vi "UDP_Test.vi"() -> ()   [LabVIEW 2016]
uses:
  SerialSupport/Serial - Settings.ctl
  SerialSupport/Serial - XON-XOFF Characters.ctl
  SerialSupport/Serial - ASCII Characters.ctl
  <vilib>/Instr/_visa.llb/VISA Configure Serial Port (Instr).vi
panel:
  in  "Stop":bool
  in  "Serial out":string caption="字符串输出"
  out "读取缓冲区":string
  in  "终止符":u8=10 format="%.0x"
  in  "终止符时结束写入？":bool=TRUE
  in  "VISA资源名称":refnum<visa-resource-name>="COM1"
  in  "XON/XOFF字符":T1={"XON"=enum."DC1", "XOFF"=enum."DC3"}
  in  "串口设置":T3={"波特率"=115200, "数据位"=8, "校验"=enum."None", "停止位"=10, "流控制"=0} {"流控制" items=["无"=0, "XON/XOFF"=1, "RTS/CTS"=2, "DTR/DSR"=4]; "停止位" items=["1.0"=10, "1.5"=15, "2.0"=20]; "数据位" min=5 max=8 step=1; "波特率" items=["75"=75, "110"=110, "134"=134, "150"=150, "300"=300, "600"=600, "1200"=1200, "1800"=1800, "2400"=2400, "4800"=4800, "7200"=7200, "9600"=9600, "14400"=14400, "19200"=19200, "28800"=28800, "38400"=38400, "56000"=56000, "57600"=57600, "115200"=115200, "128000"=128000, "230400"=230400]}
  in  "终止符时结束读取？":bool=TRUE
  out "响应":string
  in  "读数":u32=1000
  in  "读取":bool
  in  "停止 2":bool
  in  "x":dbl
  in  "string out":string caption="字符串输出"
  in  "停止":bool
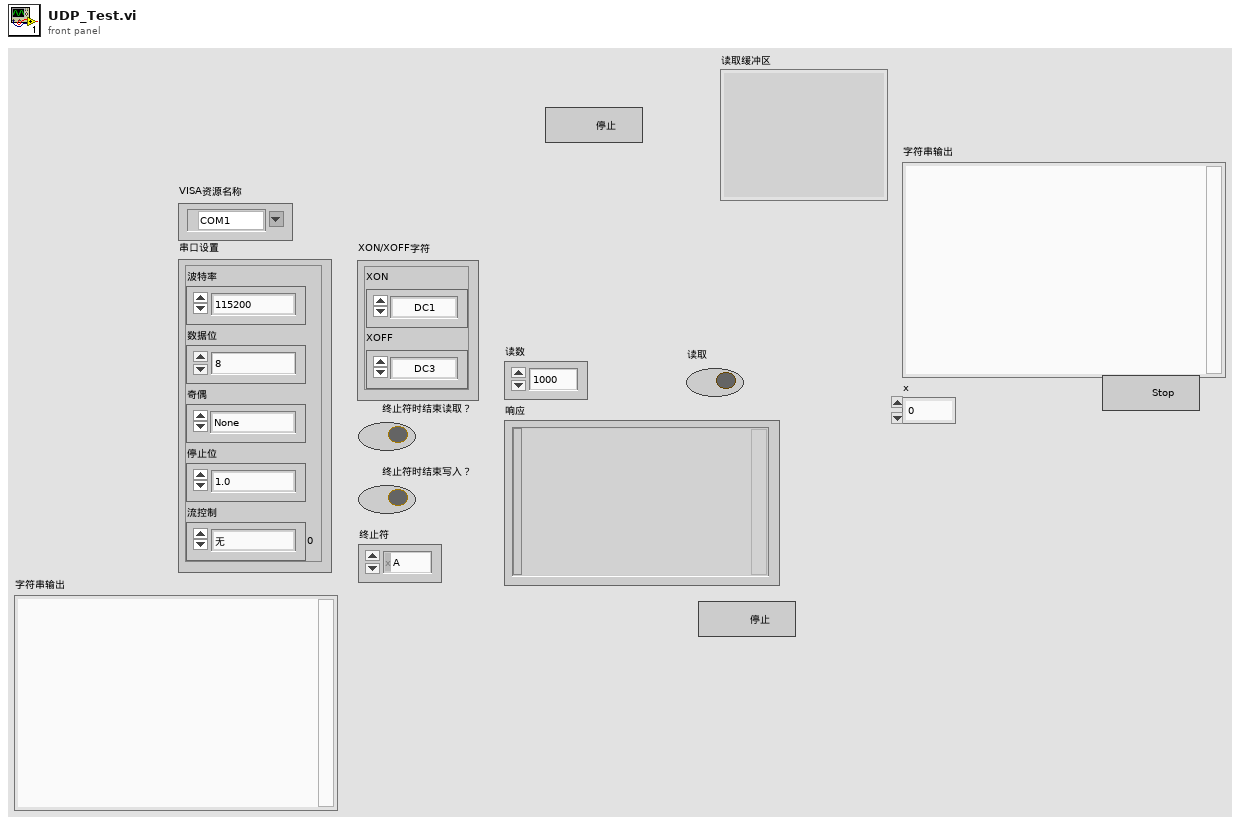
[diagram p1: front panel]
types:
  T1 = typedef "Serial - XON-XOFF Characters.ctl" = cluster{"XON":T2, "XOFF":T2}
  T2 = typedef "Serial - ASCII Characters.ctl" = enum16{"NUL", "SOH", "STX", "ETX", "EOT", "ENQ", "ACK", "BEL", "BS", "HT", "LF", "VT", "FF", "CR", "SO", "SI", "DLE", "DC1", "DC2", "DC3", "DC4", "NAK", "SYN", "ETB", "CAN", "EM", "SUB", "ESC", "FS", "GS", "RS", "US", "SP", "!", "\"", "#", "$", "%", "&", "'", "(", ")", "*", "+", ",", "- (-)", ".", "/", "0", "1", "2", "3", "4", "5", "6", "7", "8", "9", ":", ";", "<", "=", ">", "?", "@", "A", "B", "C", "D", "E", "F", "G", "H", "I", "J", "K", "L", "M", "N", "O", "P", "Q", "R", "S", "T", "U", "V", "W", "X", "Y", "Z", "[", "\\", "]", "^", "_", "`", "a", "b", "c", "d", "e", "f", "g", "h", "i", "j", "k", "l", "m", "n", "o", "p", "q", "r", "s", "t", "u", "v", "w", "x", "y", "z", "{", "|", "}", "~"}
  T3 = typedef "Serial - Settings.ctl" = cluster{"波特率":u32, "数据位":u16, "校验":enum16{"None", "Odd", "Even", "Mark", "Space"}, "停止位":u16, "流控制":u16}
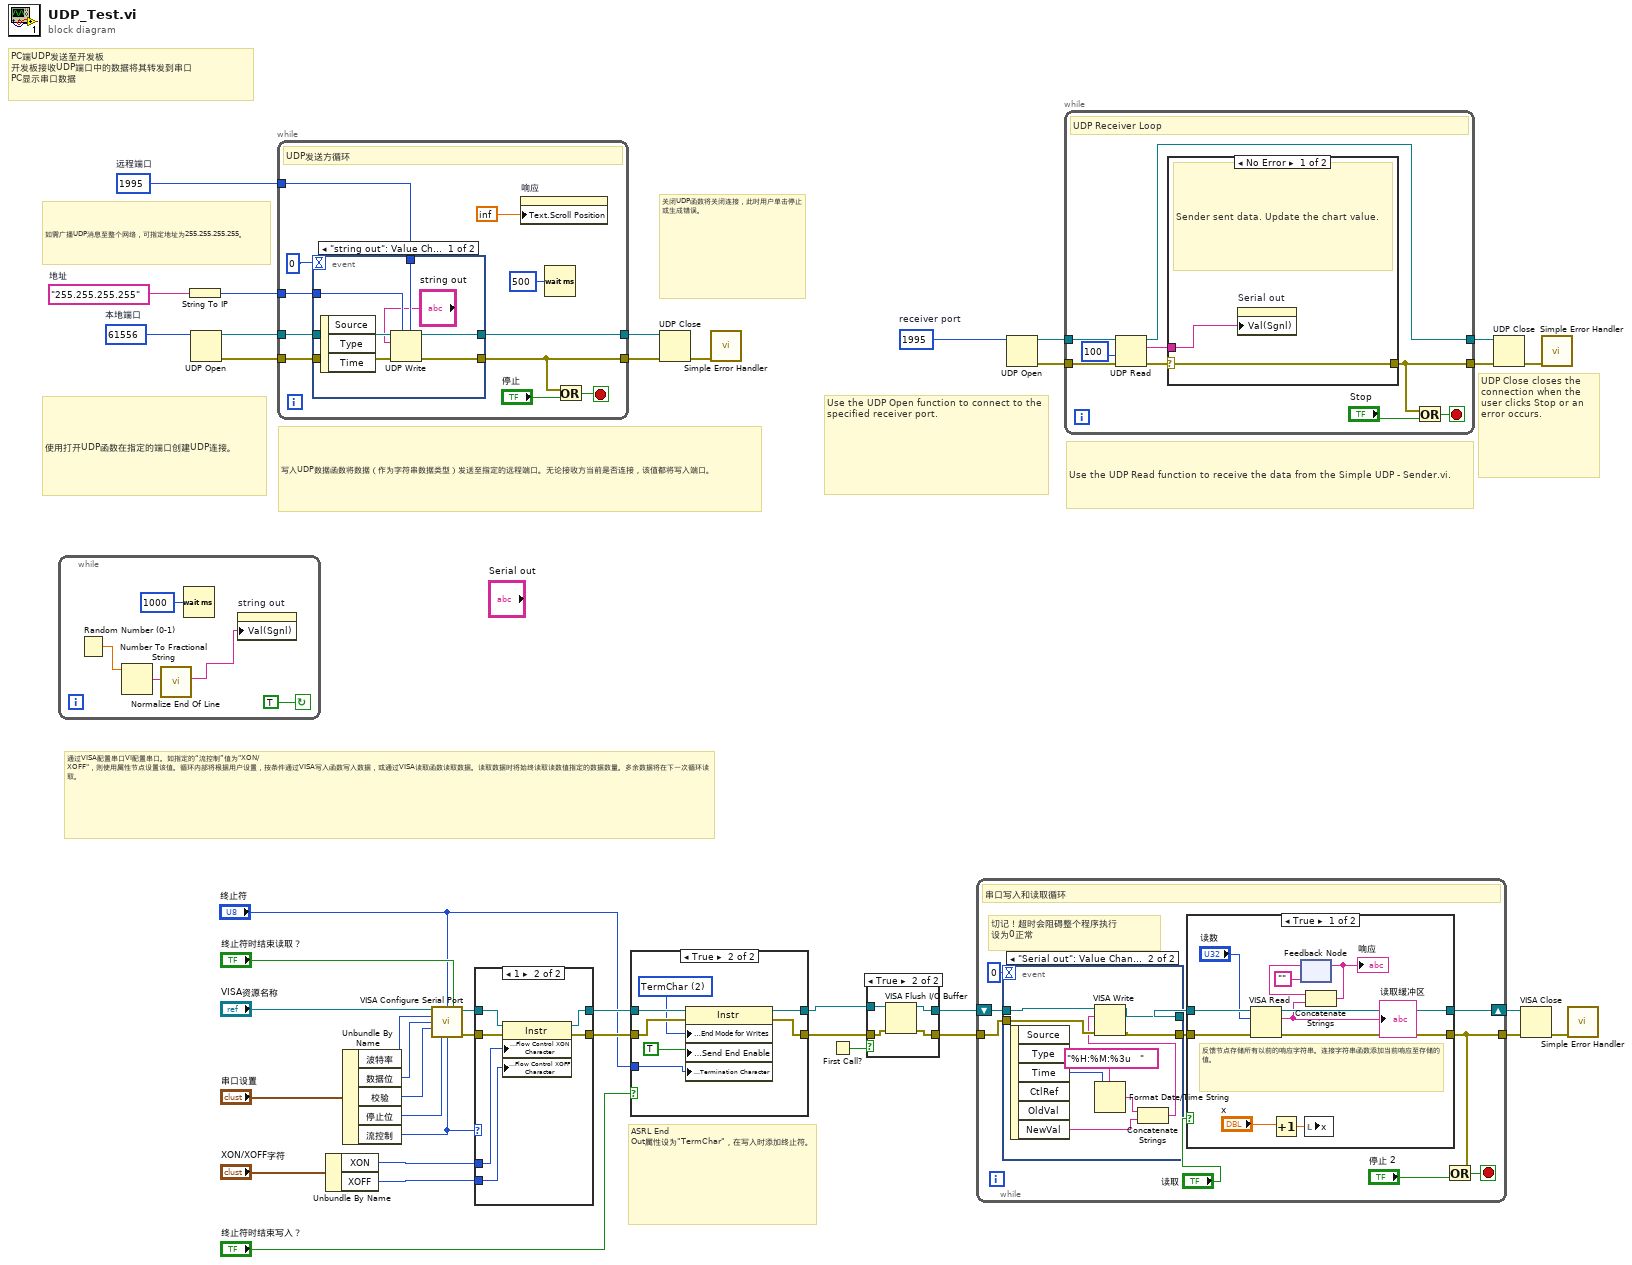
[diagram p0: block diagram]
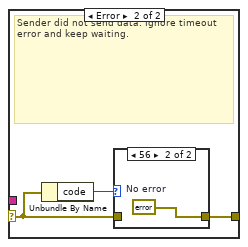
[diagram p2: hidden frame]
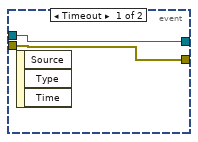
[diagram p7: hidden frame]
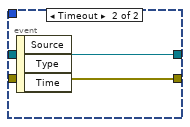
[diagram p9: hidden frame]
diagram:
  w6 = u16 1995  # receiver port
  w32 = u16 1995  # 远程端口
  w33 = u16 61556  # 本地端口
  w38 = "255.255.255.255"  # 地址
  # "UDP Close closes the connection when the user clicks Stop or an error occurs."
  # "Use the UDP Open function to connect to the specified receiver port."
  # "Use the UDP Read function to receive the data from the Simple UDP - Sender.vi."
  # "PC端UDP发送至开发板\n开发板接收UDP端口中的数据将其转发到串口\nPC显示串口数据"
  # "ASRL End Out属性设为\"TermChar\"，在写入时添加终止符。"
  # "通过VISA配置串口VI配置串口。如指定的“流控制”值为\"XON/XOFF\"，则使用属性节点设置该值。循环内部将根据用户设置，按条件通过VISA写入函数写入数据，或通过VISA读取函数读取数据。读取数据时将始终读取读数值指定的数据数量。多余数据将在下一次循环读取。"
  # "如需广播UDP消息至整个网络，可指定地址为255.255.255.255。"
  # "关闭UDP函数将关闭连接，此时用户单击停止或生成错误。"
  # "写入UDP数据函数将数据（作为字符串数据类型）发送至指定的远程端口。无论接收方当前是否连接，该值都将写入端口。"
  # "使用打开UDP函数在指定的端口创建UDP连接。"
  n1 = while {
    stop <- TRUE continue-if-true
    n2 = Random Number (0-1)() -> (number: 0 to 1=w44:dbl)
    n3 = Number To Fractional String(number=w44) -> (F-format string=w43:string)  [unwired: 3 in]
    n4 = call <vilib>:"Normalize End Of Line.vi"("string in"=w43) -> ("string out"=w41:string)  [unwired: 7 in]
    n5 = Wait (ms)(milliseconds to wait=u32 1000 ("等待时间（毫秒）")) -> ()  [unwired: 1 out]
    n6 = property on="string out" class="Str"("Val(Sgnl)"=w41) -> ()  [unwired: 2 in, 2 out]
  }
  n7 = String To IP(1:w38) -> (0:w36:u32)
  n8 = UDP Open(11:w33) -> (port=w35:refnum<k16>, 0:w34:errorcluster)  [unwired: 4 in, 1 out]
  n9 = while {
    tunnel: [w51] -> w39
    tunnel: w35 -> [w56]
    tunnel: w34 -> [w55]
    tunnel: [w52] -> w40
    tunnel: w36 -> [w50]
    tunnel: w32 -> [w48]
    stop <- w54 stop-if-true
    # "UDP发送方循环"
    n10 = event shown="[0] \"string out\": Value Change" {
      selector: _ -> [_ _]
      dyn-events: _ -> [_ _]
      timeout: 0 -> [_ _]
      tunnel: w56 -> [w63 w65]
      tunnel: w55 -> [w62 w64]
      tunnel: [w61 w65] -> w52
      tunnel: [w60 w64] -> w51
      tunnel: w50 -> [w59 _]
      tunnel: w48 -> [w58 _]
      event "string out": Value Change {
        n11 = event-data() -> ()  [unwired: 1 in, 3 out]
        n12 = UDP Write(address=w59, port or service name=w58, connection ID=w63, data in="string out", 8:w62) -> (error out=w60:errorcluster, 3:w61:refnum<k16>)  [unwired: 1 in]
      }
      event Timeout {
        n13 = event-data() -> ()  [unwired: 1 in, 3 out]
      }
    }
    n14 = property on="响应" class="Str"("Text.Scroll Position"=inf) -> ()  [unwired: 2 in, 2 out]
    n15 = Wait (ms)(milliseconds to wait=u32 500) -> ()  [unwired: 1 out]
    n16 = Or(x=w51, y="停止") -> (x .or. y?=w54:bool)
  }
  n17 = Unbundle By Name("XON/XOFF字符") -> ("XON"=w17:T2, "XOFF"=w16:T2)
  n18 = Unbundle By Name("串口设置") -> ("波特率"=w24:u32, "数据位"=w25:u16, "校验"=w26:enum16{"None", "Odd", "Even", "Mark", "Space"}, "停止位"=w27:u16, "流控制"=w18:u16)
  n19 = call-poly "VISA Configure Serial Port"("VISA resource name"="VISA资源名称", "termination char\n(0xA = '\\n' = LF)"="终止符", "Enable Termination\nChar (T)"="终止符时结束读取？", "baud rate (9600)"=w24, "data bits (8)"=w25, "parity (0:none)"=w26, "stop bits (10: 1 bit)"=w27, "flow control (0:none)"=w18) -> ("VISA resource name out"=w28:refnum<visa-resource-name>, "error out"=w29:errorcluster)  [unwired: 2 in, 4 out]
  n20 = case shown="1" w18 {
    tunnel: [w66 w73] -> w15
    tunnel: [w67 w72] -> w14
    tunnel: w29 -> [w66 w71]
    tunnel: w28 -> [w67 w70]
    tunnel: w17 -> [_ w69]
    tunnel: w16 -> [_ w68]
    frame Default {
    }
    frame 1 {
      n21 = property class="Instr"(reference=w70, error in=w71, "Serial Settings:Flow Control XON Character"=w69, "Serial Settings:Flow Control XOFF Character"=w68) -> (reference out=w72:refnum<visa-resource-name>, error out=w73:errorcluster)
    }
  }
  n22 = case shown="True" "终止符时结束写入？" {
    tunnel: w14 -> [w74 w82]
    tunnel: w15 -> [w75 w81]
    tunnel: [w74 w80] -> w11
    tunnel: [w75 w79] -> w10
    tunnel: "终止符" -> [_ w77]
    frame False {
    }
    frame True {
      w78 = u16 2 items=["None", "LastBit", "TermChar", "Break"] ("Serial Settings:Serial End Mode for Writes")
      n23 = property class="Instr"(reference=w82, error in=w81, "Serial Settings:End Mode for Writes"=w78, "Message Based Settings:Send End Enable"=TRUE, "Message Based Settings:Termination Character"=w77) -> (reference out=w80:refnum<visa-resource-name>, error out=w79:errorcluster)
    }
  }
  n24 = UDP Close(connection ID=w40, 8:w39) -> (error out=w37:errorcluster)  [unwired: 1 out]
  n25 = call <vilib>:"Simple Error Handler.vi"("error in (no error)"=w37) -> ()  [unwired: 4 in, 5 out]
  n26 = First Call?() -> (First Call?: T/F=w7:bool)
  n27 = case shown="True" w7 {
    tunnel: w11 -> [w84 w88]
    tunnel: w10 -> [w83 w87]
    tunnel: [w84 w86] -> w9
    tunnel: [w83 w85] -> w8
    frame False {
    }
    frame True {
      n28 = VISA Flush I/O Buffer(VISA resource name=w88, error in (no error)=w87) -> (VISA resource name out=w86:refnum<visa-resource-name>, error out=w85:errorcluster)  [unwired: 1 in]
    }
  }
  n29 = while {
    shift-right: [w98] -> w19
    shift-left: w9 -> [w91]
    tunnel: w8 -> [w93]
    tunnel: [w95] -> w20
    stop <- w96 stop-if-true
    # "切记！超时会阻碍整个程序执行\n设为0正常"
    # "串口写入和读取循环"
    n30 = event shown="[1] \"Serial out\": Value Change" {
      selector: _ -> [_ _]
      dyn-events: _ -> [_ _]
      timeout: 0 -> [_ _]
      tunnel: w93 -> [w99 w109]
      tunnel: [w99 w108] -> w92
      tunnel: w91 -> [w100 w107]
      tunnel: [w100 w106] -> w90
      event Timeout {
        n31 = event-data() -> ()  [unwired: 1 in, 3 out]
      }
      event "Serial out": Value Change {
        n32 = event-data() -> ("Time"=w105:u32, "NewVal"=w103:string)  [unwired: 1 in, 4 out]
        n33 = Format Date/Time String(time format string (%c)="%H:%M:%3u   " ("时间格式字符串(%c)"), seconds (now)=w105) -> (date/time string=w102:string)  [unwired: 1 in]
        n34 = Concatenate Strings(w102, w103) -> (w101:string)
        n35 = VISA Write(VISA resource name=w107, write buffer=w101, error in (no error)=w109) -> (VISA resource name out=w106:refnum<visa-resource-name>, error out=w108:errorcluster)  [unwired: 1 out]
      }
    }
    n36 = case shown="True" "读取" {
      tunnel: [w118 w122] -> w98
      tunnel: w90 -> [w120 w122]
      tunnel: [w116 w121] -> w95
      tunnel: w92 -> [w119 w121]
      frame True {
        # "反馈节点存储所有以前的响应字符串。连接字符串函数添加当前响应至存储的值。"
        n37 = VISA Read(VISA resource name=w120, byte count="读数", error in (no error)=w119) -> (VISA resource name out=w118:refnum<visa-resource-name>, read buffer=w115:string, error out=w116:errorcluster)  [unwired: 1 out]
        "读取缓冲区" <- w115
        n38 = Increment(x="x") -> (x+1=w110:dbl)
        n39 = feedback #1("") -> (w114:string)
        n40 = local write "x"(w110) -> ()
        n41 = Concatenate Strings(w114, w115) -> (w113:string)
        "响应" <- w113
        n42 = feedback-in #1(w113) -> ()
      }
      frame False {
      }
    }
    n43 = Or(x=w95, y="停止 2") -> (x .or. y?=w96:bool)
  }
  n44 = UDP Open(11:w6) -> (port=w5:refnum<k16>, 0:w4:errorcluster)  [unwired: 4 in, 1 out]
  n45 = while {
    tunnel: w5 -> [w131]
    tunnel: [w123] -> w1
    tunnel: w4 -> [w128]
    tunnel: [w124] -> w3
    stop <- w129 stop-if-true
    # "UDP Receiver Loop"
    n46 = UDP Read(connection ID=w131, timeout ms (25000)=100, 8:w128) -> (data out=w126:string, error out=w125:errorcluster, 3:w123:refnum<k16>)  [unwired: 3 out]
    n47 = case shown="No Error" w125 {
      selector: w125 -> [w133 w135]
      tunnel: w126 -> [w132 _]
      tunnel: [w133 w134] -> w124
      frame No Error {
        # "Sender sent data. Update the chart value."
        n48 = property on="Serial out" class="Str"("Val(Sgnl)"=w132) -> ()  [unwired: 2 in, 2 out]
      }
      frame Error {
        # "Sender did not send data. Ignore timeout error and keep waiting."
        n49 = Unbundle By Name(w135) -> ("code"=w136:i32)
        n50 = case shown="56" w136 {
          tunnel: w135 -> [w137 _]
          tunnel: [w137 w138] -> w134
          frame Default {
          }
          frame 56 {
            w138 = errorcluster {"status"=FALSE, "code"=0, "source"=""}  # No error
          }
        }
      }
    }
    n51 = Or(x=w124, y="Stop") -> (x .or. y?=w129:bool)
  }
  n52 = UDP Close(connection ID=w1, 8:w3) -> (error out=w2:errorcluster)  [unwired: 1 out]
  n53 = VISA Close(VISA resource name=w19, error in (no error)=w20) -> (error out=w21:errorcluster)
  n54 = call <vilib>:"Simple Error Handler.vi"("error in (no error)"=w2) -> ()  [unwired: 1 in, 8 out]
  n55 = call <vilib>:"Simple Error Handler.vi"("error in (no error)"=w21) -> ()  [unwired: 1 in, 8 out]
